vi "WriteParent.vi"(8 "error in":errorcluster, 10 "parent":T1, 11 "node in":refnum<class "CEF_Node.lvclass">) -> (0 "error out":errorcluster, 3 "node out":refnum<class "CEF_Node.lvclass">)   [LabVIEW 2025, in "CEF.lvlib" / "CEF_Node.lvclass"]
doc: "Copyright 2017 National Instruments Corporation\n\nLicensed under the Apache License, Version 2.0 (the \"License\"); you may not use this file except in compliance with the License. You may obtain a copy of the License at http://www.apache.org/licenses/LICENSE-2.0\nUnless required by applicable law or agreed to in writing, software distributed under the License is distributed on an \"AS IS\" BASIS, WITHOUT WARRANTIES OR CONDITIONS OF ANY KIND, either express or implied. See the License for the specific language governing permissions and limitations under the License."
uses:
  CEF_Node.lvclass
  NodeRef.ctl
  CEF_Node.lvclass/CEF_Node.ctl
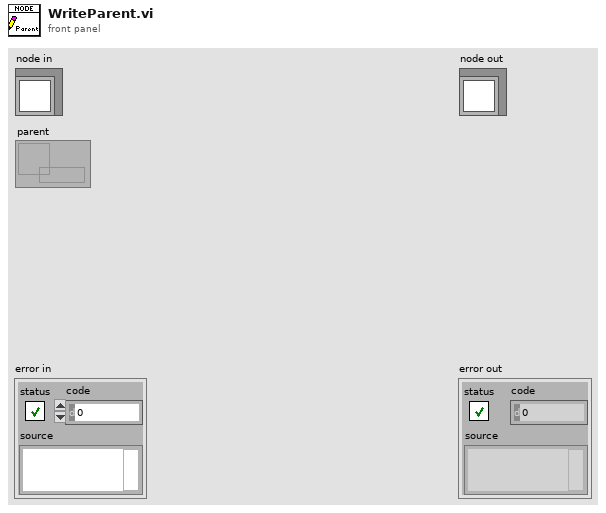
[diagram p1: front panel]
types:
  T1 = typedef "CEF.lvlib/CEF_Node.lvclass/NodeRef.ctl" = refnum<data-value>
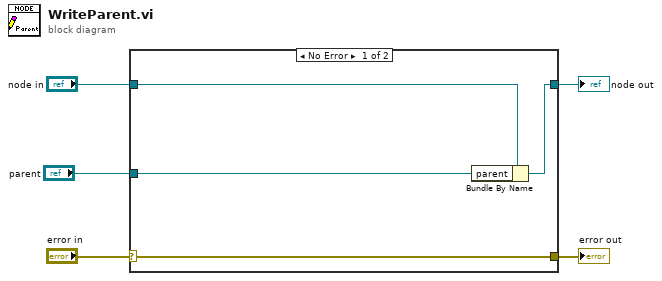
[diagram p0: block diagram]
diagram:
  n1 = case shown="No Error" "error in" {
    selector: "error in" -> [w9 w10]
    tunnel: [w9 w10] -> w4
    tunnel: [w7 w11] -> w2
    tunnel: "node in" -> [w8 w11]
    tunnel: "parent" -> [w6 _]
    frame No Error {
      n2 = Bundle By Name(cluster=w8, "parent"=w6) -> (w7:refnum<class "CEF_Node.lvclass">)
    }
    frame Error {
    }
  }
  "error out" <- w4
  "node out" <- w2
